vi "non_FPGA_VI_v1.vi"() -> ()   [LabVIEW 2020]
uses:
  c5c29772-c0b0-45e0-ac49-cc5077cfdad3.vi
  <vilib>/Array/Sort 2D Array - Pop Stack.vi
  <vilib>/Array/Sort 2D Array - Push Stack.vi
  c5c29772-c0b0-45e0-ac49-cc5077cfdad3.vi/269d4b3b-47f5-49e3-8884-44851e4dd9d5.vi
  c5c29772-c0b0-45e0-ac49-cc5077cfdad3.vi/6d99389c-673d-4efb-bf33-19b32bcf4cf8.vi
  <vilib>/Analysis/NI_AALBase.lvlib
panel:
  out "sorted array":sgl[](graph)
  out "sorted array index":i32[](array[numeric])
  out "sorted array img":sgl[](array[numeric])
  out "sorted array real":sgl[](array[numeric])
  out "sorted 2D array":dbl[][](array[numeric])
  out "appended array":dbl[][](array[numeric])
  out "sorted array":dbl[](array[numeric])
  out "uniform white noise":dbl[](array[numeric])
  out "array input":dbl[](graph)
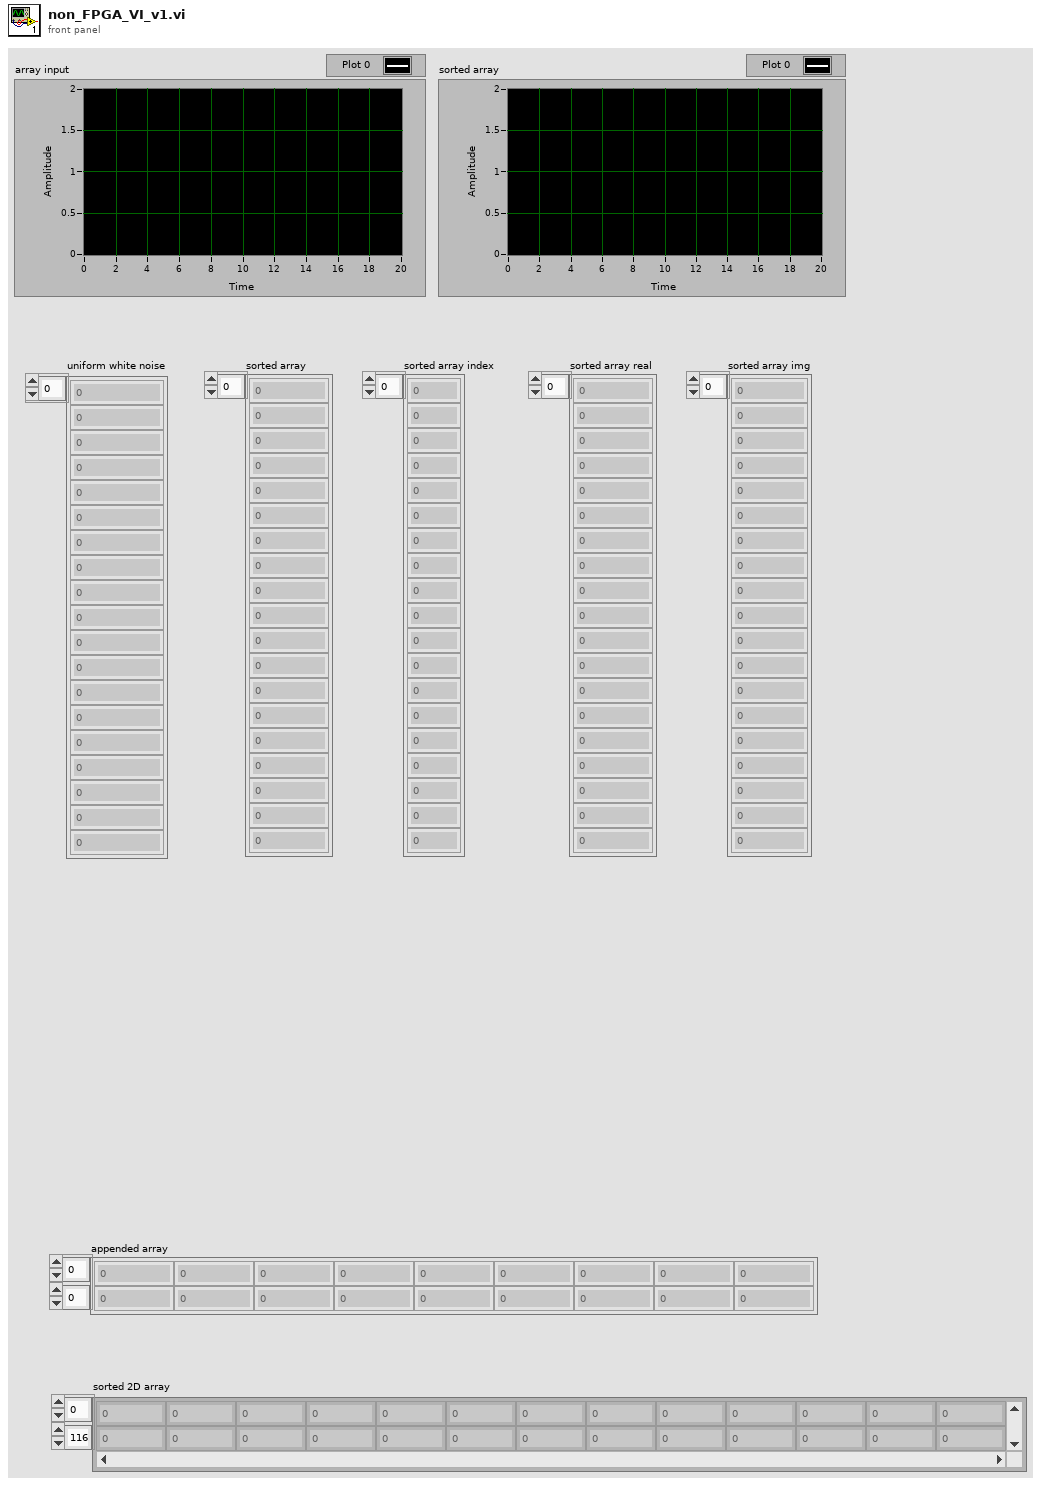
[diagram p1: front panel]
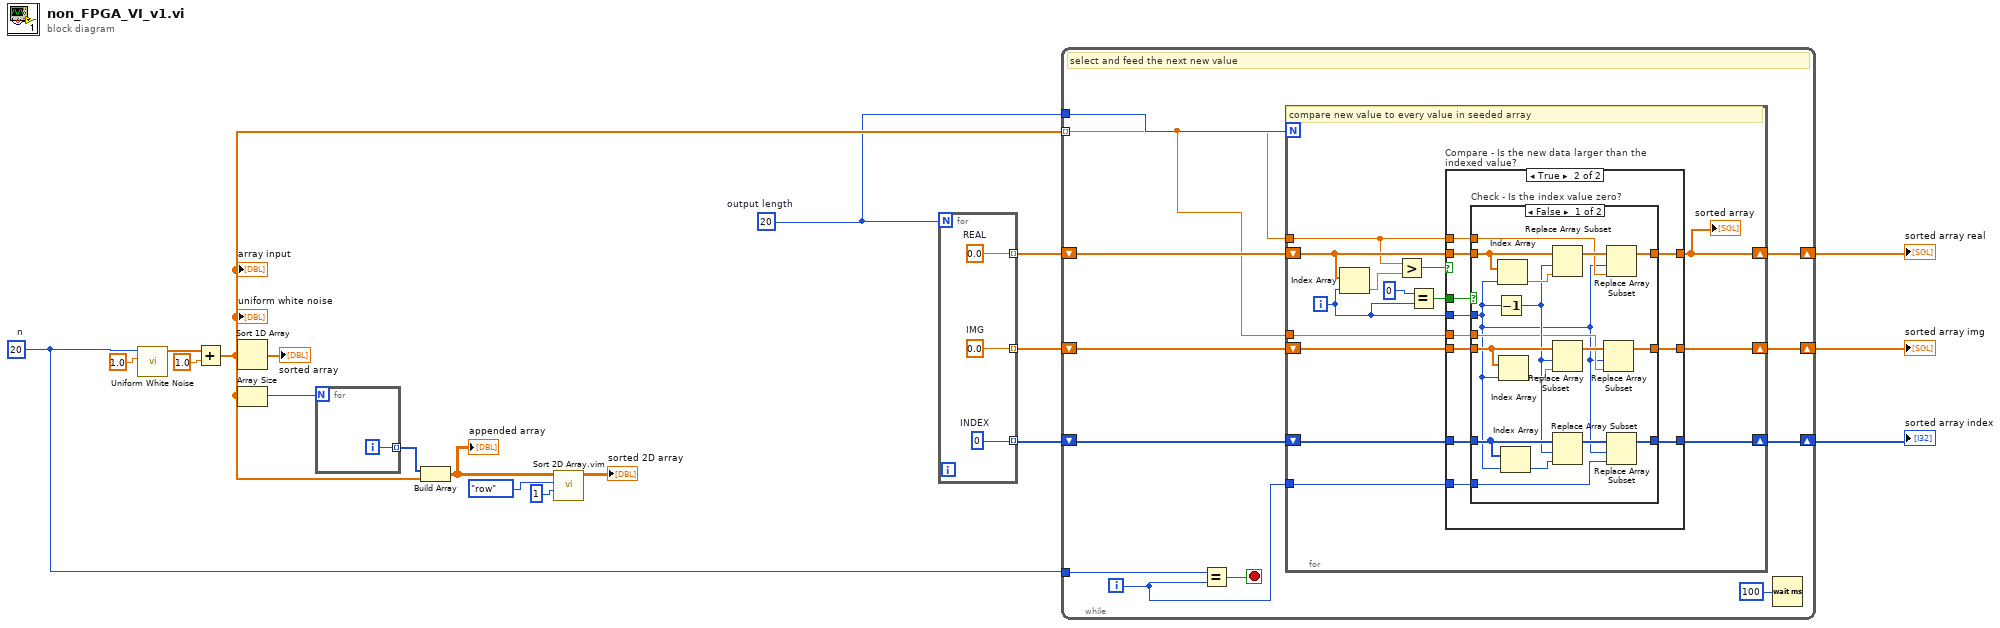
[diagram p0: block diagram]
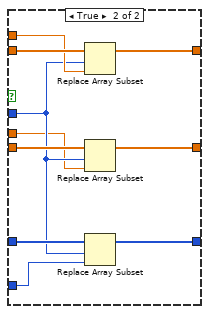
[diagram p3: hidden frame]
diagram:
  w2 = 20  # output length
  w4 = 20  # n
  n1 = call <vilib>:"Uniform White Noise.vi"("amplitude"=1.0, "samples"=w4) -> ("uniform white noise"=w15:dbl[])  [unwired: 8 in, 1 out]
  n2 = Add(x=w15, y=1.0 ("amplitude")) -> (x+y=w3:dbl[])
  "array input" <- w3
  "uniform white noise" <- w3
  n3 = Sort 1D Array(array=w3) -> (sorted array=→"sorted array":dbl[])
  n4 = Array Size(array=w3) -> (size(s)=w16:i32)
  n5 = for {
    N: w16 -> [_]
    tunnel: [w20] -> w14 mode=indexing
    i -> [w20]
  }
  n6 = Build Array(w14, w3) -> (w13:dbl[][])
  "appended array" <- w13
  n7 = call "Sort 2D Array.vim"("index"=1, "dimension to index (column)"=enum16{"column", "row"}."row", "2D array"=w13) -> ("sorted 2D array"=→"sorted 2D array":dbl[][])  [unwired: 7 in, 1 out]
  n8 = for {
    N: w2 -> [_]
    tunnel: [w23] -> w8 mode=indexing
    tunnel: [w22] -> w9 mode=indexing
    tunnel: [w21] -> w7 mode=indexing
    w21 = sgl 0.0  # IMG
    w22 = 0  # INDEX
    w23 = sgl 0.0  # REAL
  }
  n9 = while {
    shift-right: [w26] -> w1
    shift-left: w8 -> [w35]
    shift-right: [w34] -> w6
    shift-left: w9 -> [w33]
    tunnel: w4 -> [w31]
    shift-right: [w29] -> w5
    shift-left: w7 -> [w28]
    tunnel: w3 -> [w24] mode=indexing
    tunnel: w2 -> [w27]
    i -> [w32]
    stop <- w30 stop-if-true
    # "select and feed the next new value"
    n10 = Equal?(x=w31, y=w32) -> (x = y?=w30:bool)
    n11 = for {
      N: w27 -> [_]
      tunnel: w24 -> [w46]
      shift-right: [w45] -> w26
      shift-left: w35 -> [w47]
      tunnel: w32 -> [w43]
      shift-right: [w41] -> w34
      shift-left: w33 -> [w42]
      shift-right: [w38] -> w29
      shift-left: w28 -> [w37]
      tunnel: w24 -> [w36]
      i -> [w44]
      # "compare new value to every value in seeded array"
      n12 = Index Array(array=w47, index=w44) -> (element=w49:sgl)
      n13 = Greater?(x=w46, y=w49) -> (0:w48:bool)
      n14 = Equal?(x=0, y=w44) -> (x = y?=w39:bool)
      n15 = case "Compare - Is the new data larger than the indexed value?" shown="True" w48 {
        tunnel: w47 -> [w52 w62]
        tunnel: w39 -> [_ w63]
        tunnel: w46 -> [_ w61]
        tunnel: w44 -> [_ w60]
        tunnel: [w52 w59] -> w45
        tunnel: w43 -> [_ w58]
        tunnel: w42 -> [w51 w57]
        tunnel: [w51 w56] -> w41
        tunnel: [w50 w55] -> w38
        tunnel: w37 -> [w50 w54]
        tunnel: w36 -> [_ w53]
        frame False {
        }
        frame True {
          n16 = case "Check - Is the index value zero?" shown="False" w63 {
            tunnel: w62 -> [w80 w90]
            tunnel: w61 -> [w77 w89]
            tunnel: w60 -> [w64 w83]
            tunnel: [w76 w88] -> w59
            tunnel: w58 -> [w71 w87]
            tunnel: w57 -> [w73 w86]
            tunnel: [w72 w85] -> w56
            tunnel: [w66 w81] -> w55
            tunnel: w54 -> [w70 w84]
            tunnel: w53 -> [w65 w82]
            frame False {
              n17 = Decrement(x=w64) -> (x-1=w68:i32)
              n18 = Index Array(array=w80, index=w64) -> (element=w79:sgl)
              n19 = Index Array(array=w70, index=w64) -> (element=w69:sgl)
              n20 = Index Array(array=w73, index=w64) -> (element=w75:i32)
              n21 = Replace Array Subset(array=w80, new element=w79, index=w68) -> (w78:sgl[])
              n22 = Replace Array Subset(array=w70, new element=w69, index=w68) -> (w67:sgl[])
              n23 = Replace Array Subset(array=w73, new element=w75, index=w68) -> (w74:i32[])
              n24 = Replace Array Subset(array=w67, new element=w65, index=w64) -> (w66:sgl[])
              n25 = Replace Array Subset(array=w78, new element=w77, index=w64) -> (w76:sgl[])
              n26 = Replace Array Subset(array=w74, new element=w71, index=w64) -> (w72:i32[])
            }
            frame True {
              n27 = Replace Array Subset(array=w90, new element=w89, index=w83) -> (w88:sgl[])
              n28 = Replace Array Subset(array=w84, new element=w82, index=w83) -> (w81:sgl[])
              n29 = Replace Array Subset(array=w86, new element=w87, index=w83) -> (w85:i32[])
            }
          }
        }
      }
      "sorted array" <- w45
    }
    n30 = Wait (ms)(milliseconds to wait=u32 100) -> ()  [unwired: 1 out]
  }
  "sorted array real" <- w1
  "sorted array img" <- w5
  "sorted array index" <- w6
